vi "Datos gita.vi"() -> ()   [LabVIEW 2017]
uses:
  <vilib>/Utility/file.llb/Write Delimited Spreadsheet (DBL).vi
panel:
  in  "Numeric":i32
  out "Theta Pot_min":dbl
  out "Theta Pot_max":dbl
  out "Pot_min":dbl
  out "Pot_max":dbl
  out "path 2":path
  out "Potencia vs Angulo":cluster{"Y":dbl[], "Y":dbl[]}[](graph)
  in  "Archivo de texto":path
  out "theta":dbl
  in  "Angulo inicial":dbl
  in  "Paso motor":dbl
  out "path":path
  out "concatenated string":string
  out "Reconocimiento 3":T1(plugin-control)
  out "Lectura":string
  out "Imagen orginal 2":T1(plugin-control)
  in  "imagenes":path
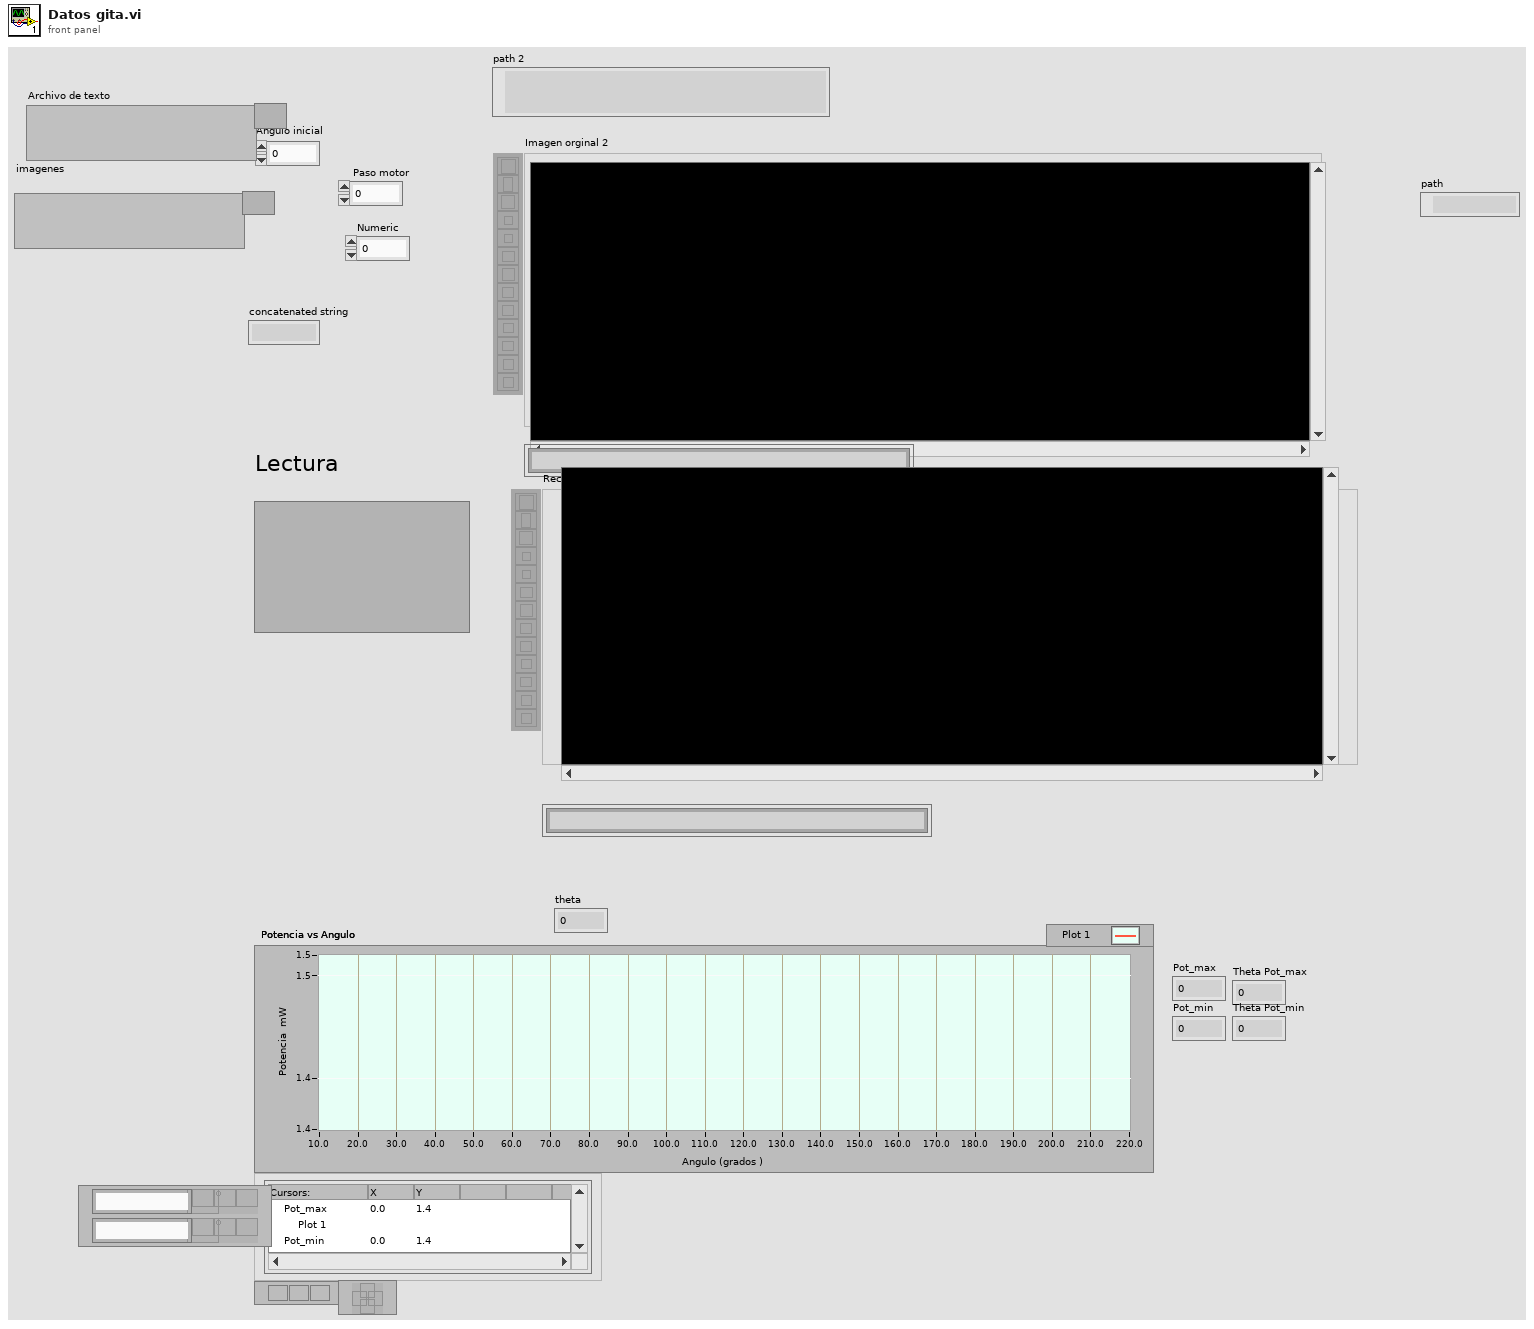
[diagram p1: front panel]
types:
  T1 = typedef "IMAQ Image.ctl" = refnum<image>
  T2 = enum16{"open", "replace", "create", "open or create", "replace or create", "replace or create with confirmation"}
  T3 = typedef "Image Type" = u32
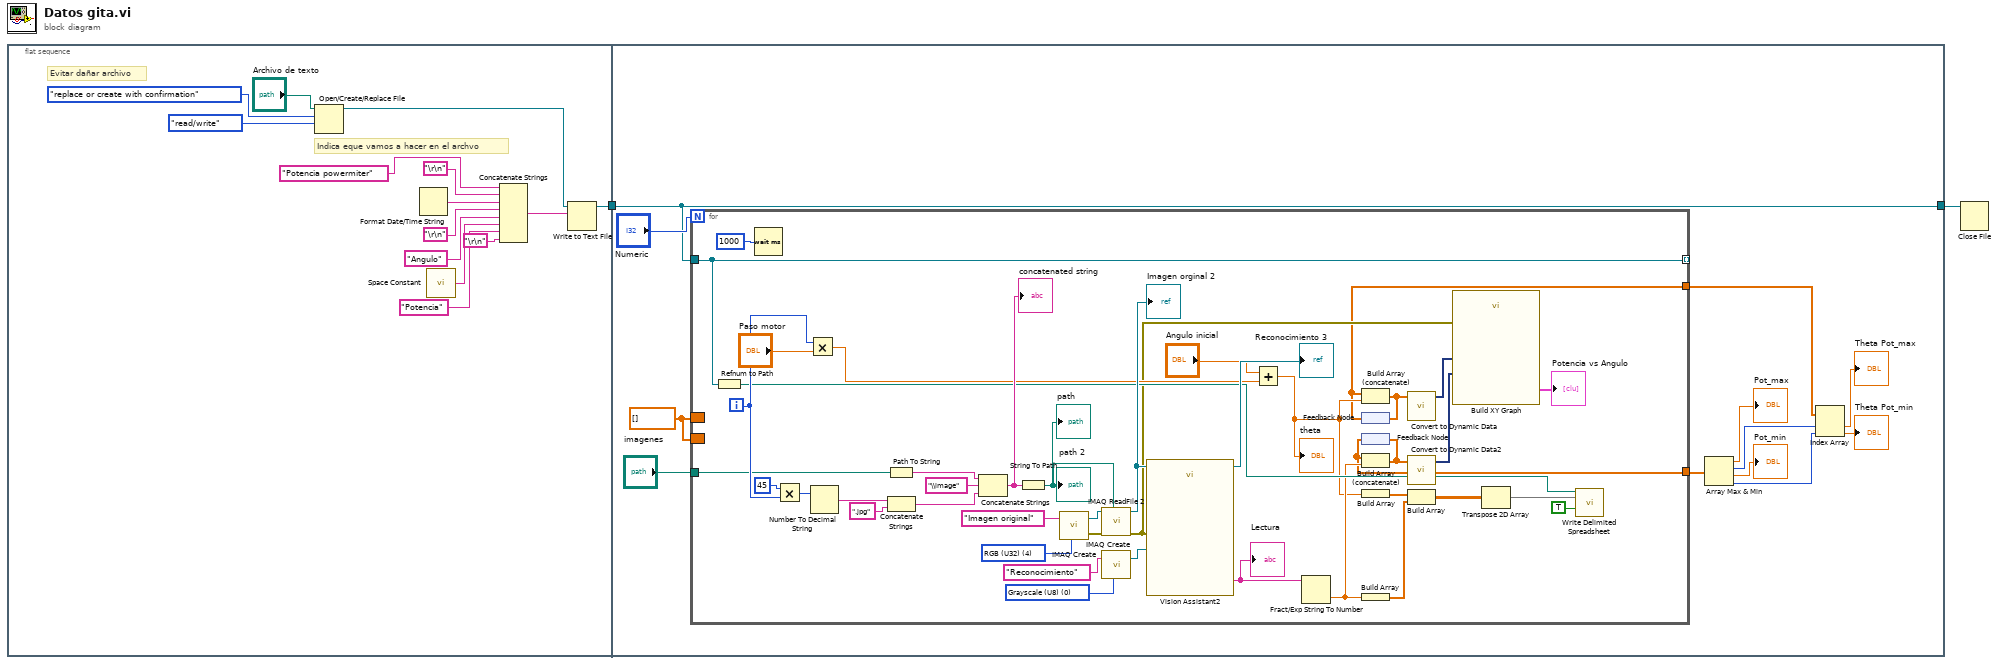
[diagram p0: block diagram]
diagram:
  n1 = flat-sequence {
    tunnel: [w4] -> w2
    tunnel: w2 -> [w27]
    tunnel: [w27] -> w1
    frame #0 {
      # "Indica eque vamos a hacer en el archvo"
      # "Evitar dañar archivo"
      n2 = Open/Create/Replace File(file path (use dialog)="Archivo de texto", operation (0:open)=T2."replace or create with confirmation", access (0:read/write)=enum16{"read/write", "read-only", "write-only"}."read/write") -> (refnum out=w7:refnum<file>)  [unwired: 3 in, 2 out]
      n3 = Format Date/Time String() -> (date/time string=w14:string)  [unwired: 3 in]
      n4 = call <vilib>:"Space Constant.vi"() -> ("String"=w16:string)
      n5 = Concatenate Strings("Potencia powermiter", "\r\n", w14, "\r\n", "Angulo", w16, "Potencia", "\r\n") -> (w15:string)
      n6 = Write to Text File(file (use dialog)=w7, text=w15) -> (refnum out=w4:refnum<file>)  [unwired: 2 in, 2 out]
    }
    frame #1 {
      w25 = dbl[] []
      n7 = for {
        N: "Numeric" -> [_]
        border: w25 -> [_]
        tunnel: "imagenes" -> [w46]
        tunnel: w27 -> [w43]
        tunnel: [w43] -> _ mode=indexing
        border: w25 -> [_]
        tunnel: [w30] -> w24
        tunnel: [w29] -> w23
        i -> [w51]
        w63 = T3 0 items=["Grayscale (U8)", "Grayscale (I16)", "Grayscale (SGL)", "Complex (CSG)", "RGB (U32)", "HSL (U32)", "RGB (U64)", "Grayscale (U16)"] ("Image Type")
        w64 = T3 4 items=["Grayscale (U8)", "Grayscale (I16)", "Grayscale (SGL)", "Complex (CSG)", "RGB (U32)", "HSL (U32)", "RGB (U64)", "Grayscale (U16)"] ("Image Type")
        n8 = Refnum to Path(1:w43) -> (0:w45:path)
        n9 = Wait (ms)(milliseconds to wait=u32 1000) -> ()  [unwired: 1 out]
        n10 = Multiply(x=45, y=w51) -> (x*y=w58:i32)
        n11 = Multiply(x=w51, y="Paso motor") -> (x*y=w49:dbl)
        n12 = Number To Decimal String(number=w58) -> (decimal integer string=w54:string)  [unwired: 1 in]
        n13 = Path To String(path=w46) -> (string=w61:string)
        n14 = Concatenate Strings(w54, ".jpg" ("string")) -> (w52:string)
        n15 = Concatenate Strings(w61, "\\image", w52) -> (w57:string)
        "concatenated string" <- w57
        n16 = String To Path(string=w57) -> (path=w56:path)
        "path" <- w56
        "path 2" <- w56
        n17 = call "IMAQ Create"("Image Name"="Imagen original", "Image Type"=w64) -> ("New Image"=w69:T1, "error out"=w68:errorcluster)  [unwired: 3 in]
        n18 = call "IMAQ ReadFile 2"("File Path"=w56, "error in (no error)"=w68, "Image"=w69) -> ("error out"=w37:errorcluster, "Image Out"=w67:T1)  [unwired: 4 in, 3 out]
        "Imagen orginal 2" <- w67
        n19 = call "IMAQ Create"("Image Name"="Reconocimiento", "Image Type"=w63) -> ("New Image"=w65:T1)  [unwired: 3 in, 1 out]
        n20 = call "Vision Assistant2"("Image In"=w67, "Image Dst"=w65, "error in"=w37) -> ("Image Out"=→"Reconocimiento 3":T1, "String (OCR/OCV 3)"=w47:string)  [unwired: 22 in, 1 out]
        "Lectura" <- w47
        n21 = Add(x="Angulo inicial", y=w49) -> (x+y=w31:dbl)
        "theta" <- w31
        n22 = Fract/Exp String To Number(string=w47) -> (number=w36:dbl)  [unwired: 3 in, 1 out]
        n23 = feedback #1() -> (w30:dbl[])
        n24 = Build Array (concatenate)(w30, w31) -> (w35:dbl[])
        n25 = feedback-in #1(w35) -> ()
        n26 = feedback #2() -> (w29:dbl[])
        n27 = Build Array (concatenate)(w29, w36) -> (w33:dbl[])
        n28 = feedback-in #2(w33) -> ()
        n29 = Build Array(w31) -> (w40:dbl[])
        n30 = Build Array(w36) -> (w39:dbl[])
        n31 = call "Convert to Dynamic Data"("Array"=w35) -> ("Dynamic Data Type"=w34:dynamicdata)  [unwired: 3 in]
        n32 = call "Convert to Dynamic Data2"("Array"=w33) -> ("Dynamic Data Type"=w32:dynamicdata)  [unwired: 3 in]
        n33 = Build Array(w40, w39) -> (w42:dbl[][])
        n34 = call "Build XY Graph"("error in (no error)"=w37, "Y Input"=w32, "X Input"=w34) -> ("XY Graph"=→"Potencia vs Angulo":cluster{"X":dbl[], "Y":dbl[]}[])  [unwired: 7 in, 1 out]
        n35 = Transpose 2D Array(2D array=w42) -> (transposed array=w41:dbl[][])
        n36 = call-poly <vilib>:"Write Delimited Spreadsheet.vi"("file path (dialog if empty)"=w45, "2D data"=w41, "append to file? (new file:F)"=TRUE) -> ()  [unwired: 11 in, 2 out]
      }
      n37 = Array Max & Min(array=w23) -> (max value=→"Pot_max":dbl, max index (indices)=w22:i32, min value=→"Pot_min":dbl, min index (indices)=w21:i32)
      n38 = Index Array(array=w24, index #1=w22, index #2=w21) -> (element #1=→"Theta Pot_max":dbl, element #2=→"Theta Pot_min":dbl)
    }
  }
  n39 = Close File(refnum=w1) -> ()  [unwired: 1 in, 2 out]
